vi "Sys config window-Set wavelengths ring.vi"(9 "Laser wavelength (nm)":u16, 11 "System Config window refs":T1) -> (1 "Wavelength already exists":bool)   [LabVIEW 2020]
uses:
  Typedefs/HW config window refs cluster.ctl
  Typedefs/HW Setup tab control.ctl
  Typedefs/Control Sys HW config cluster.ctl
  Typedefs/CTRL system config.ctl
  Peripherals Control/Triggers/Typedefs/General trigger settings cluster.ctl
  Typedefs/Trigger 1 selector enum.ctl
  Typedefs/Triggers HW config.ctl
  Peripherals Control/Triggers/Typedefs/Triggers output setup.ctl
  Peripherals Control/Triggers/Typedefs/Trigger setup element cluster.ctl
  Typedefs/DAQ FPGA HW config cluster.ctl
  RIG-SPECIFIC FILES/FPGA Refs/FPGA Ref.ctl
  <vilib>/userDefined/High Color/nirio_resource_hc.ctl
  Typedefs/FPGA input type AC-DC.ctl
  Typedefs/DAQ FPGA system config.ctl
  Peripherals Control/XYZ Stage/Control/typedefs/XYZControlConfig.ctl
  Typedefs/Peripherals comms config cluster.ctl
  Typedefs/Comms Type.ctl
  Typedefs/Encoder config cluster.ctl
  Typedefs/Cam VidRec HW config setup cluster.ctl
  Typedefs/AOD Settings-distilled.ctl
  Typedefs/Laser Power Control HW config.ctl
  Typedefs/Laser 1 config cluster.ctl
  Typedefs/PreChirper 1 config cluster.ctl
  Typedefs/PreChirper constants.ctl
  Configuration code/Calibration/Globals/gl_Calibration globals.vi
panel:
  # "General Setup"
  # "Control System"
  # "Triggers"
  # "DAQ FPGA"
  # "HW Channels Setup"
  # "XYZ Stage"
  # "Encoder"
  # "redundant"
  # "redundant"
  # "redundant"
  # "redundant"
  # "Hardware Setup"
  # "CamVideo"
  # "redundant"
  # "redundant"
  # "AOL Properties"
  # "Calib. Settings"
  # "Laser Settings"
  # "PreChirper Settings"
  # "(make , model etc)"
  # "(COM Port / IP Address / service address etc.)"
  # "(Port for ethernet / channel for BT)"
  # "(make , model etc)"
  # "(COM Port / IP Address / service address etc.)"
  # "(Port for ethernet / channel for BT)"
  # "(make , model etc)"
  # "(COM Port / IP Address / service address etc.)"
  # "(Port for ethernet / channel for BT)"
  # "Thickness (mm)"
  # "X Offset"
  # "Separation (mm)"
  # "Y Offset"
  # "Centre (mm)"
  # "Timing Offset"
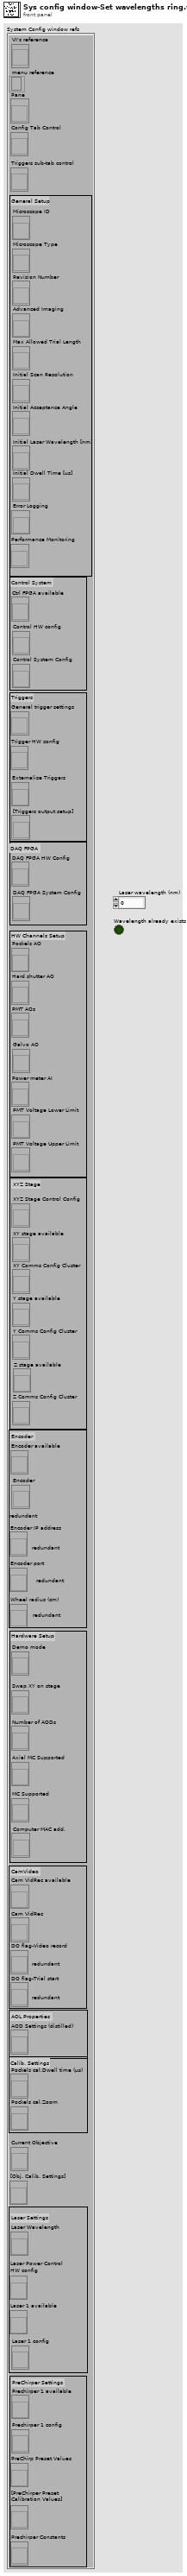
[diagram p1: front panel]
types:
  T1 = typedef "HW config window refs cluster.ctl" = cluster{"VI's reference":refnum<vi>, "menu reference":refnum<k9>, "Pane":refnum<vi>, "Config Tab Control":refnum<vi>, "Triggers sub-tab control":refnum<vi>, "Microscope ID":refnum<vi>, "Microscope Type":refnum<vi>, "Revision Number":refnum<vi>, "Advanced Imaging":refnum<vi>, "Max Allowed Trial Length":refnum<vi>, "Initial Scan Resolution":refnum<vi>, "Initial Acceptance Angle":refnum<vi>, "Initial Laser Wavelength [nm] ":refnum<vi>, "Initial Dwell Time [us]":refnum<vi>, "Error Logging":refnum<vi>, "Performance Monitoring":refnum<vi>, "Ctrl FPGA available":refnum<vi>, "Control HW config":refnum<vi>, "Control System Config":refnum<vi>, "General trigger settings":refnum<vi>, "Trigger HW config":refnum<vi>, "Externalise Triggers":refnum<vi>, "[Triggers output setup]":refnum<vi>, "DAQ FPGA HW Config":refnum<vi>, "DAQ FPGA System Config":refnum<vi>, "Pockels AO":refnum<vi>, "Hard shutter AO":refnum<vi>, "PMT AOs":refnum<vi>, "Galvo AO":refnum<vi>, "Power meter AI":refnum<vi>, "PMT Voltage Lower Limit":refnum<vi>, "PMT Voltage Upper Limit":refnum<vi>, "XYZ Stage Control Config":refnum<vi>, "XY stage available":refnum<vi>, "XY Comms Config Cluster":refnum<vi>, "Y stage available":refnum<vi>, "Y Comms Config Cluster":refnum<vi>, "Z stage available":refnum<vi>, "Z Comms Config Cluster":refnum<vi>, "Encoder available":refnum<vi>, "Encoder":refnum<vi>, "Encoder IP address":refnum<vi>, "Encoder port":refnum<vi>, "Wheel radius (cm)":refnum<vi>, "Demo mode":refnum<vi>, "Swap XY on stage":refnum<vi>, "Number of AODs":refnum<vi>, "Axial MC Supported":refnum<vi>, "MC Supported":refnum<vi>, "Computer MAC add.":refnum<vi>, "Cam VidRec available":refnum<vi>, "Cam VidRec":refnum<vi>, "DO flag-Video record":refnum<vi>, "DO flag-Trial start":refnum<vi>, "AOD Settings (distilled)":refnum<vi>, "Pockels cal.Dwell time (µs)":refnum<vi>, "Pockels cal.Zoom":refnum<vi>, "Current Objective":refnum<vi>, "[Obj. Calib. Settings]":refnum<vi>, "Laser Wavelength":refnum<vi>, "Laser Power Control \nHW config":refnum<vi>, "Laser 1 available":refnum<vi>, "Laser 1 config":refnum<vi>, "Prechirper 1 available":refnum<vi>, "Prechirper 1 config":refnum<vi>, "PreChirp Preset Values":refnum<vi>, "[PreChirper Preset \nCalibration Values]":refnum<vi>, "Prechirper Constants":refnum<vi>}
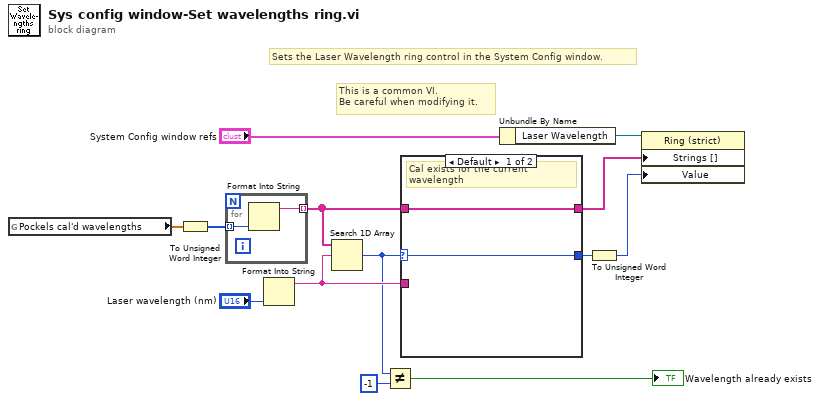
[diagram p0: block diagram]
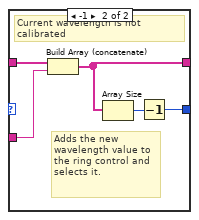
[diagram p2: hidden frame]
diagram:
  # "This is a common VI.\nBe careful when modifying it."
  # "Sets the Laser Wavelength ring control in the System Config window."
  n1 = global read "gl_Calibration globals.vi" "Pockels cal'd wavelengths"() -> (w12:dbl[])
  n2 = To Unsigned Word Integer(number=w12) -> (unsigned 16bit integer=w11:u16[])
  n3 = for {
    tunnel: w11 -> [w15] mode=indexing
    tunnel: [w14] -> w4 mode=indexing
    n4 = Format Into String(w15) -> (resulting string=w14:string)  [unwired: 3 in, 1 out]
  }
  n5 = Format Into String("Laser wavelength (nm)") -> (resulting string=w5:string)  [unwired: 3 in, 1 out]
  n6 = Search 1D Array(1D array=w4, element=w5) -> (index of element=w3:i32)  [unwired: 1 in]
  n7 = Not Equal?(x=w3, y=-1) -> (x != y?=→"Wavelength already exists":bool)
  n8 = case shown="Default" w3 {
    selector: w3 -> [w17 _]
    tunnel: [w17 w18] -> w8
    tunnel: w4 -> [w16 w21]
    tunnel: w5 -> [_ w22]
    tunnel: [w16 w20] -> w6
    frame Default {
      # "Cal exists for the current wavelength"
    }
    frame -1 {
      # "Adds the new wavelength value to the ring control and selects it."
      # "Current wavelength is not calibrated"
      n9 = Build Array (concatenate)(w21, w22) -> (w20:string[])
      n10 = Array Size(array=w20) -> (size(s)=w19:i32)
      n11 = Decrement(x=w19) -> (x-1=w18:i32)
    }
  }
  n12 = Unbundle By Name("System Config window refs") -> ("Laser Wavelength"=w7:refnum<vi>)
  n13 = To Unsigned Word Integer(number=w8) -> (unsigned 16bit integer=w9:u16)
  n14 = property on="Property Node" class="Ring (strict)"(reference=w7, "Strings []"=w6, "Value"=w9) -> ()  [unwired: 1 in, 2 out]
